vi "A-Star Search.vi"(11 "Puzzle 15-1 In":T3) -> (3 "Min Risk":i32)   [LabVIEW 2020]
uses:
  Puzzle 15-1.ctl
  Position.ctl
  Dir.ctl
  <vilib>/Utility/miscctls.llb/LVMapReplaceAction.ctl
panel:
  out "F":i32[][](array[numeric])
  out "Map":map{i32, T1[]}(c390)
  out "Open":bool[][](array[boolean])
  out "From":T2[][](array[typedef])
  out "G":i32[][](array[numeric])
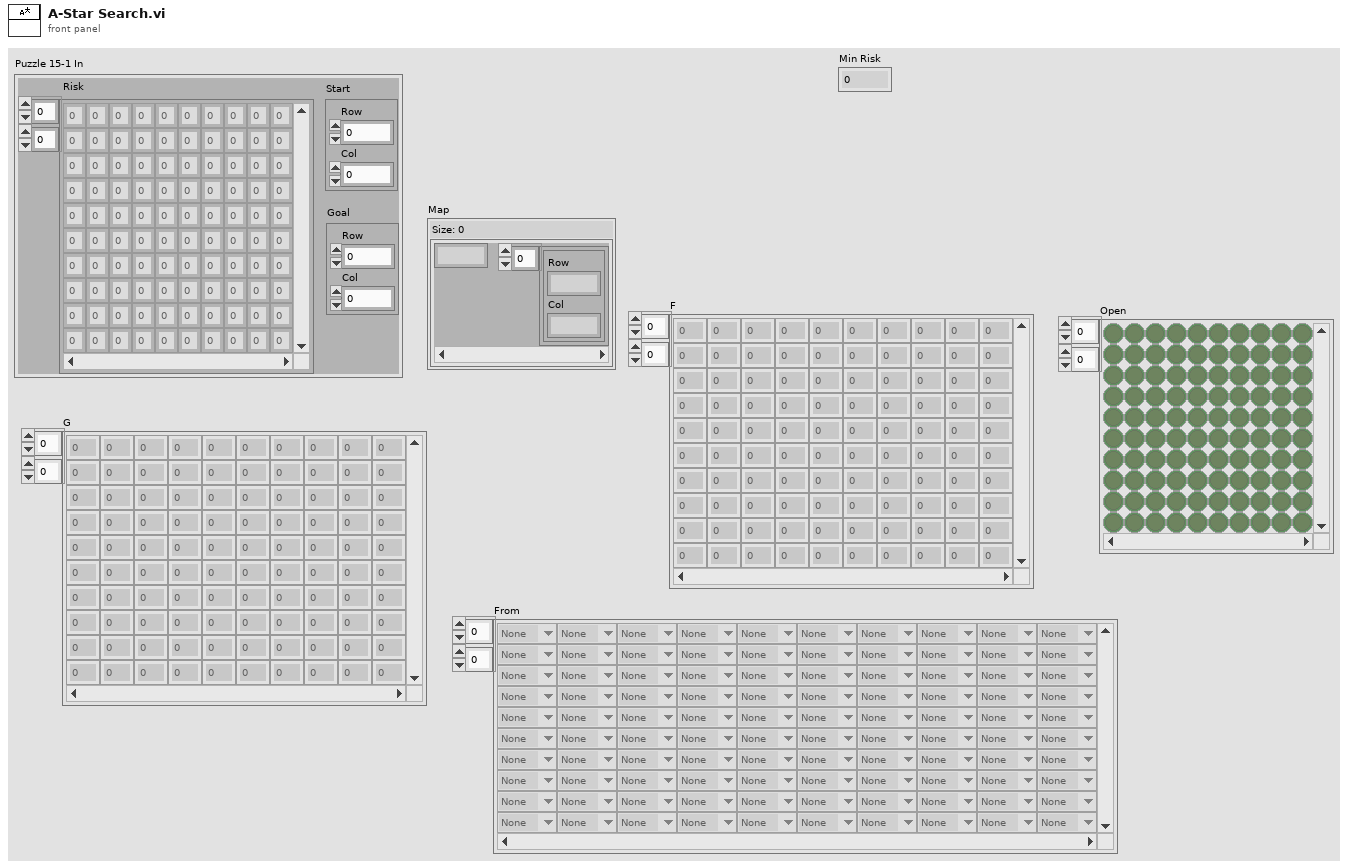
[diagram p1: front panel]
types:
  T1 = typedef "Position.ctl" = cluster{"Row":i32, "Col":i32}
  T2 = typedef "Dir.ctl" = enum16{"None", "Up", "Left", "Down", "Right"}
  T3 = typedef "Puzzle 15-1.ctl" = cluster{"Risk":i32[][], "Start":T1, "Goal":T1}
  T4 = typedef "LVMapReplaceAction.ctl" = enum32{"Modify Entry only if found", "Add or Modify Entry", "Delete Entry"}
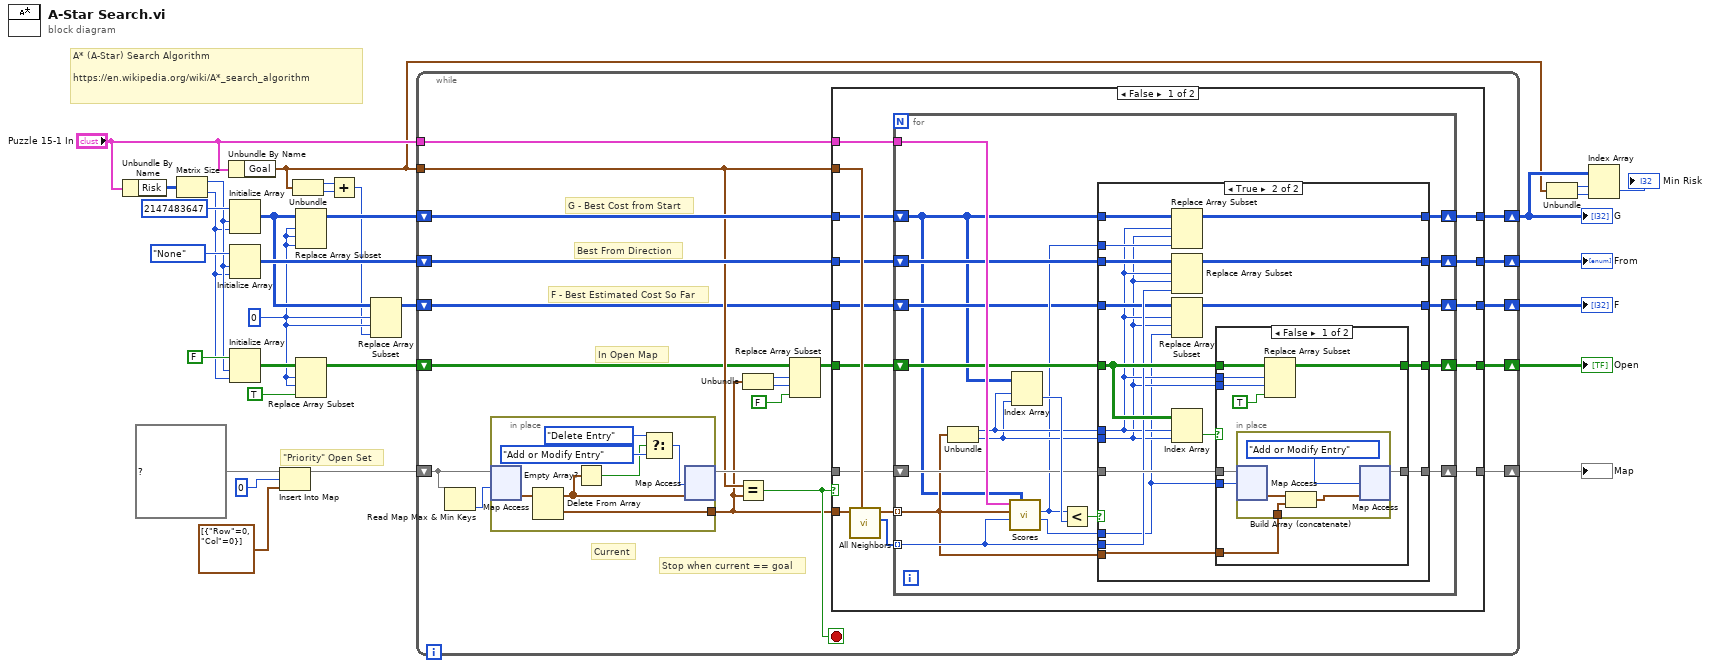
[diagram p0: block diagram]
diagram:
  w8 = 0 ("index (row)")
  # "A* (A-Star) Search Algorithm\n\nhttps://en.wikipedia.org/wiki/A*_search_algorithm"
  # "\"Priority\" Open Set"
  n1 = Unbundle By Name("Puzzle 15-1 In") -> ("Risk"=w26:i32[][])
  n2 = Matrix Size(0:w26) -> (1:w20:i32, 2:w19:i32)
  n3 = Unbundle By Name("Puzzle 15-1 In") -> ("Goal"=w2:T1)
  n4 = Initialize Array(2147483647, w20, w19) -> (w9:i32[][])
  n5 = Initialize Array(Dir."None" ("Dir"), w20, w19) -> (w23:T2[][])
  n6 = Initialize Array(FALSE, w20, w19) -> (w18:bool[][])
  n7 = Insert Into Map(map in=map{i32, T1[]} {} ("Open Map"), key=0, value=T1[] [{"Row"=0, "Col"=0}]) -> (map out=w25:map{i32, T1[]})  [unwired: 2 out]
  n8 = Unbundle(w2) -> ("Row"=w12:i32, "Col"=w11:i32)
  n9 = Replace Array Subset(array=w9, new element=w8, index (row)=w8, index (col)=w8) -> (w24:i32[][])
  n10 = Replace Array Subset(array=w18, new element=TRUE ("new element/subarray"), index (row)=w8, index (col)=w8) -> (w16:bool[][])
  n11 = Add(x=w12, y=w11) -> (x+y=w7:i32)
  n12 = Replace Array Subset(array=w9, new element=w7, index (row)=w8, index (col)=w8) -> (w10:i32[][])
  n13 = while {
    shift-right: [w47] -> w13
    shift-left: w25 -> [w51]
    shift-right: [w43] -> w5
    shift-left: w24 -> [w44]
    tunnel: "Puzzle 15-1 In" -> [w42]
    shift-right: [w45] -> w15
    shift-left: w23 -> [w46]
    tunnel: w2 -> [w41]
    shift-right: [w40] -> w14
    shift-left: w16 -> [w39]
    shift-right: [w33] -> w6
    shift-left: w10 -> [w32]
    stop <- w49 stop-if-true
    # "F - Best Estimated Cost So Far"
    # "Stop when current == goal"
    # "In Open Map"
    # "Best From Direction"
    # "G - Best Cost from Start"
    # "Current"
    n14 = Read Map Max & Min Keys(11:w51) -> (1:w50:i32)  [unwired: 1 out]
    n15 = in-place {
      in-place-border: [w57] -> w37
      n16 = in-place-map #1(w51, w50) -> (w58:T1[])  [unwired: 1 in, 1 out]
      n17 = Delete From Array(array=w58) -> (deleted portion=w57:T1, array with subset deleted=w56:T1[])  [unwired: 2 in]
      n18 = Empty Array?(array=w56) -> (empty?=w53:bool)
      n19 = Select(t=LVMapReplaceAction."Delete Entry" ("action"), s=w53, f=LVMapReplaceAction."Add or Modify Entry" ("action")) -> (s? t:f=w52:T4)
      n20 = in-place-map #1(w56, w52) -> (w48:map{i32, T1[]})  [unwired: 2 out]
    }
    n21 = Equal?(x=w41, y=w37) -> (x = y?=w49:bool)
    n22 = Unbundle(w37) -> ("Row"=w36:i32, "Col"=w35:i32)
    n23 = Replace Array Subset(array=w39, new element=FALSE ("new element/subarray"), index (row)=w36, index (col)=w35) -> (w38:bool[][])
    n24 = case shown="False" w49 {
      tunnel: w48 -> [w69 w134]
      tunnel: [w65 w134] -> w47
      tunnel: w46 -> [w70 w133]
      tunnel: [w66 w133] -> w45
      tunnel: w44 -> [w71 w132]
      tunnel: [w67 w132] -> w43
      tunnel: w42 -> [w64 _]
      tunnel: w37 -> [w73 _]
      tunnel: w41 -> [w72 _]
      tunnel: w38 -> [w62 w131]
      tunnel: [w61 w131] -> w40
      tunnel: [w60 w130] -> w33
      tunnel: w32 -> [w59 w130]
      frame False {
        n25 = call "All Neighbors.vi"("Goal"=w72, "Position"=w73) -> ("Froms"=w63:T2[], "All Neighbors"=w68:T1[])  [unwired: 7 in, 1 out]
        n26 = for {
          shift-right: [w80] -> w67
          shift-left: w71 -> [w74]
          shift-right: [w79] -> w66
          shift-left: w70 -> [w89]
          shift-right: [w77] -> w65
          shift-left: w69 -> [w87]
          tunnel: w68 -> [w81] mode=indexing
          tunnel: w64 -> [w92]
          tunnel: w63 -> [w88] mode=indexing
          shift-right: [w78] -> w61
          shift-left: w62 -> [w86]
          shift-right: [w75] -> w60
          shift-left: w59 -> [w76]
          n27 = Unbundle(w81) -> ("Row"=w85:i32, "Col"=w84:i32)
          n28 = call "Scores.vi"("G"=w74, "From"=w88, "Position"=w81, "Puzzle 15-1"=w92) -> ("F(n)"=w82:i32, "G(n)"=w83:i32)  [unwired: 4 in, 2 out]
          n29 = Index Array(array=w74, index (row)=w85, index (col)=w84) -> (element=w91:i32)
          n30 = Less?(x=w83, y=w91) -> (x < y?=w90:bool)
          n31 = case shown="True" w90 {
            tunnel: w89 -> [w96 w107]
            tunnel: w74 -> [w97 w109]
            tunnel: w88 -> [_ w106]
            tunnel: w87 -> [w94 w111]
            tunnel: w86 -> [w95 w113]
            tunnel: [w97 w104] -> w80
            tunnel: [w96 w105] -> w79
            tunnel: [w95 w112] -> w78
            tunnel: [w94 w110] -> w77
            tunnel: w85 -> [_ w100]
            tunnel: w84 -> [_ w99]
            tunnel: w83 -> [_ w108]
            tunnel: w82 -> [_ w98]
            tunnel: w81 -> [_ w103]
            tunnel: [w93 w102] -> w75
            tunnel: w76 -> [w93 w101]
            frame False {
            }
            frame True {
              n32 = Replace Array Subset(array=w109, new element=w108, index (row)=w100, index (col)=w99) -> (w104:i32[][])
              n33 = Replace Array Subset(array=w107, new element=w106, index (row)=w100, index (col)=w99) -> (w105:T2[][])
              n34 = Replace Array Subset(array=w101, new element=w98, index (row)=w100, index (col)=w99) -> (w102:i32[][])
              n35 = Index Array(array=w113, index (row)=w100, index (col)=w99) -> (element=w114:bool)
              n36 = case shown="False" w114 {
                tunnel: w113 -> [w120 w129]
                tunnel: [w119 w129] -> w112
                tunnel: w111 -> [w123 w128]
                tunnel: [w121 w128] -> w110
                tunnel: w103 -> [w122 _]
                tunnel: w100 -> [w118 _]
                tunnel: w99 -> [w117 _]
                tunnel: w98 -> [w115 _]
                frame False {
                  n37 = in-place {
                    in-place-border: w122 -> [w126]
                    n38 = in-place-map #2(w123, w115) -> (w125:T1[])  [unwired: 1 in, 1 out]
                    n39 = Build Array (concatenate)(w125, w126) -> (w124:T1[])
                    n40 = in-place-map #2(w124, LVMapReplaceAction."Add or Modify Entry" ("action")) -> (w121:map{i32, T1[]})  [unwired: 2 out]
                  }
                  n41 = Replace Array Subset(array=w120, new element=TRUE ("new element/subarray"), index (row)=w118, index (col)=w117) -> (w119:bool[][])
                }
                frame True {
                }
              }
            }
          }
        }
      }
      frame True {
      }
    }
  }
  "G" <- w5
  "From" <- w15
  "Open" <- w14
  "Map" <- w13
  "F" <- w6
  n42 = Unbundle(w2) -> ("Row"=w4:i32, "Col"=w3:i32)
  n43 = Index Array(array=w5, index (row)=w4, index (col)=w3) -> (element=→"Min Risk":i32)
